vi "RunMe (Test Launcher).vi"() -> ()   [LabVIEW 2013, in "Test Runner.BrokenTest.lvclass"]
uses:
  Test Runner.BrokenTest.lvclass
  classes/Test Runner/Test Runner.lvclass
panel:
  out "error out":errorcluster
  # "RUN ME.\n\nThis VI is an example of a Test Suite created as a Test Runner extension"
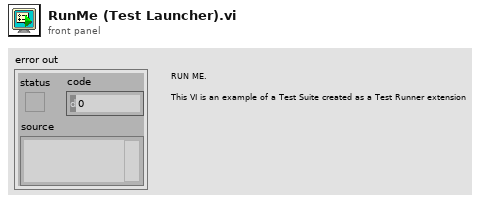
[diagram p1: front panel]
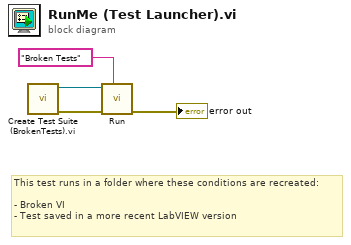
[diagram p0: block diagram]
diagram:
  # "This test runs in a folder where these conditions are recreated: \n\n- Broken VI\n- Test saved in a more recent LabVIEW version"
  n1 = call "Create Test Suite (BrokenTests).vi.vi"() -> ("error out"=w3:errorcluster, "Test Runner.BrokenTests"=w4:refnum<class "Test Runner.BrokenTest.lvclass">)  [unwired: 10 in]
  n2 = call "Run.vi"("Name"="Broken Tests", "error in (no error)"=w3, "Test Runner in"=w4) -> ("error out"=→"error out":errorcluster)  [unwired: 6 in, 2 out]
